vi "DIAdem Process Datasheet Request.vi"(5 "error in (no error)":errorcluster, 7 "DIAdem Queue":T1, 8 "DIAdem Reference":T3) -> (0 "error out":errorcluster, 2 "Script Result":string, 3 "dup DIAdem Reference":T3)   [LabVIEW 2011]
uses:
  <vilib>/ExportToExcel/DIAdem Reference.ctl
  DIAdem Daemon Queue.ctl
  DIAdem Daemon Script Type.ctl
  datasheet script data.ctl
  Addons/internet/utils/keyedarr.llb/Keyed Array.ctl
  Addons/DIAdem/DIAdem.llb/DIAdem String Variable Set.vi
  Addons/DIAdem/DIAdem.llb/DIAdem String Variable Get.vi
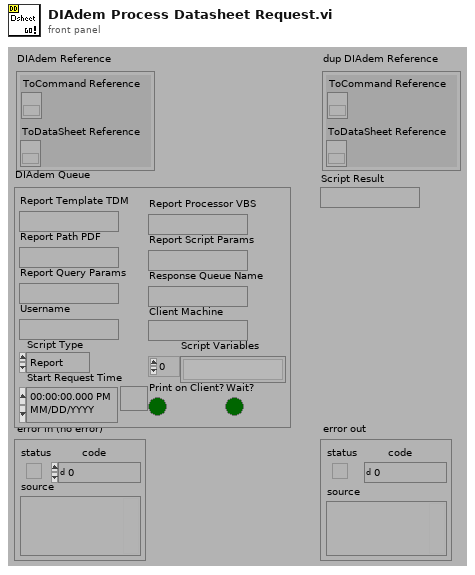
[diagram p1: front panel]
types:
  T1 = typedef "DIAdem Daemon Queue.ctl" = cluster{"Report Template TDM":path, "Report Processor VBS":path, "Report Path PDF":path, "Report Script Params":string, "Username":string, "Script Type":T2, "Report Query Params":string, "Client Machine":string, "Print on Client?":bool, "Response Queue Name":string, "Script Variables":string[], "Start Request Time":timestamp, "Wait?":bool}
  T2 = typedef "DIAdem Daemon Script Type.ctl" = enum16{"Report", "Query", "Script", "Datasheet", "Append", "Restart", "Stop"}
  T3 = typedef "DIAdem Reference.ctl" = cluster{"ToCommand Reference":refnum<k7>, "ToDataSheet Reference":refnum<k7>}
  T4 = typedef "datasheet script data.ctl" = cluster{"Script":path, "Parameters":T5, "sxTemplateId":string, "Estimate":i32}
  T5 = typedef "Keyed Array.ctl" = cluster{"keys":string[], "values":string[]}
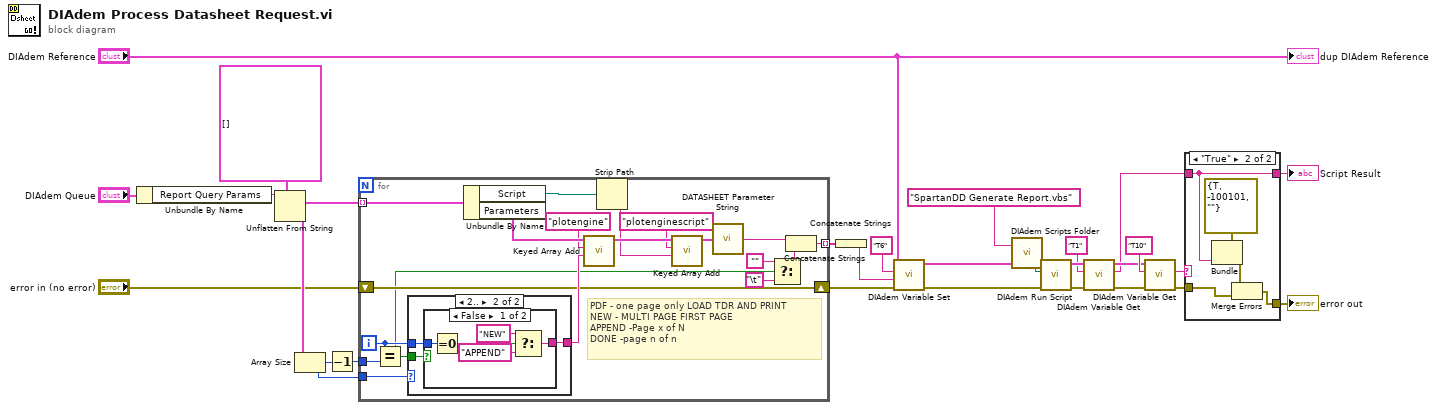
[diagram p0: block diagram]
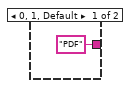
[diagram p3: hidden frame]
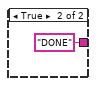
[diagram p4: hidden frame]
diagram:
  n1 = Unbundle By Name("DIAdem Queue") -> ("Report Query Params"=w26:string)
  n2 = Unflatten From String(type=T4[] [], binary string=w26) -> (value=w25:T4[])  [unwired: 1 in, 4 out]
  n3 = Array Size(array=w25) -> (size(s)=w24:i32)
  n4 = Decrement(x=w24) -> (x-1=w11:i32)
  n5 = for {
    tunnel: w25 -> [w45] mode=indexing
    shift-right: [w30] -> w23
    shift-left: "error in (no error)" -> [w30]
    tunnel: w11 -> [w46]
    tunnel: w24 -> [w44]
    tunnel: [w31] -> w22 mode=indexing
    i -> [w29]
    # "PDF - one page only LOAD TDR AND PRINT\nNEW - MULTI PAGE FIRST PAGE\nAPPEND -Page x of N\nDONE -page n of n"
    n6 = Equal?(x=w29, y=w46) -> (x = y?=w28:bool)
    n7 = case shown="2.." w44 {
      tunnel: w28 -> [_ w50]
      tunnel: ["PDF" w49] -> w40
      tunnel: w29 -> [_ w48]
      frame 0, 1, Default {
      }
      frame 2.. {
        n8 = case shown="False" w50 {
          tunnel: [w55 "DONE"] -> w49
          tunnel: w48 -> [w51 _]
          frame False {
            n9 = Equal To 0?(x=w51) -> (x = 0?=w52:bool)
            n10 = Select(t="NEW", s=w52, f="APPEND") -> (s? t:f=w55:string)
          }
          frame True {
          }
        }
      }
    }
    n11 = Unbundle By Name(w45) -> ("Script"=w43:path, "Parameters"=w42:T5)
    n12 = call "Keyed Array Add.vi"("value"=w40, "key"="plotengine", "array in"=w42) -> ("array out"=w38:T5)  [unwired: 1 in, 3 out]
    n13 = Strip Path(path=w43) -> (name=w37:string)  [unwired: 1 out]
    n14 = call "Keyed Array Add.vi"("value"=w37, "key"="plotenginescript", "array in"=w38) -> ("array out"=w39:T5)  [unwired: 1 in, 3 out]
    n15 = call "DATASHEET Parameter String.vi"("params"=w39) -> ("url-encoded param string"=w35:string)
    n16 = Select(t="", s=w28, f="\t") -> (s? t:f=w32:string)
    n17 = Concatenate Strings(w35, w32) -> (w31:string)
  }
  n18 = Concatenate Strings(w22) -> (w10:string)
  n19 = call-poly "DIAdem Variable Set.vi"("error in (no error)"=w23, "Value"=w10, "Variable Name"="T6", "DIAdem Reference"="DIAdem Reference") -> ("error out"=w16:errorcluster, "DIAdem Reference"=w17:T3)  [unwired: 6 out]
  n20 = call "DIAdem Scripts Folder.vi"("Relative Path (\"\" - Folder)"="SpartanDD Generate Report.vbs" ("Relative Path (\"\" - Folder)")) -> ("Scripts Folder"=w18:path)  [unwired: 2 out]
  n21 = call "DIAdem Run Script.vi"("error in (no error)"=w16, "script file"=w18, "DIAdem Reference"=w17) -> ("error out"=w14:errorcluster, "DIAdem Reference"=w15:T3)  [unwired: 7 out]
  n22 = call-poly "DIAdem Variable Get.vi"("error in (no error)"=w14, "Variable Name"="T1", "DIAdem Reference"=w15) -> ("error out"=w7:errorcluster, "Value"=w5:string, "DIAdem Reference"=w6:T3)  [unwired: 6 out]
  n23 = call-poly "DIAdem Variable Get.vi"("error in (no error)"=w7, "Variable Name"="T10", "DIAdem Reference"=w6) -> ("error out"=w4:errorcluster, "Value"=w2:string)  [unwired: 7 out]
  n24 = case shown="\"True\"" w2 {
    tunnel: w5 -> [w57 w59]
    tunnel: w4 -> [w58 w62]
    tunnel: [w58 w60] -> w3
    tunnel: [w57 w59] -> w1
    frame Default {
    }
    frame "True" {
      n25 = Bundle(cluster=errorcluster {"status"=TRUE, "code"=-100101, "source"=""} ("error out"), "source"=w59) -> (w61:errorcluster)  [unwired: 2 in]
      n26 = Merge Errors(w61, w62) -> (w60:errorcluster)
    }
  }
  "error out" <- w3
  "Script Result" <- w1
  "dup DIAdem Reference" <- "DIAdem Reference"
